vi "Spawn.vi"(7 "ConcreteActor":refnum<class "ConcreteActor.lvclass">) -> (4 "Error":errorcluster, 5 "ConcreteActor":refnum<class "ConcreteActor.lvclass">)   [LabVIEW 2020, in "_Template.lvlib" / "ActorTemplate.lvlib" / "{{Name}}.lvlib" / "ConcreteActor.lvclass"]
uses:
  ConcreteActor.lvclass
  ConcreteActor.lvclass/ConcreteActor.ctl
  jettl/jettl/Actor/Actor.lvclass
panel:
  # "This front panel should not be manipulated."
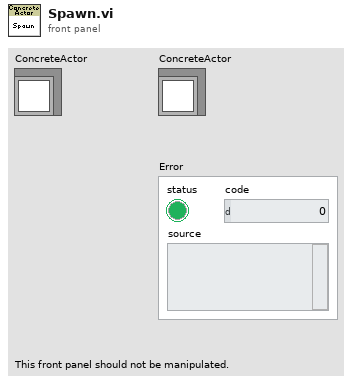
[diagram p1: front panel]
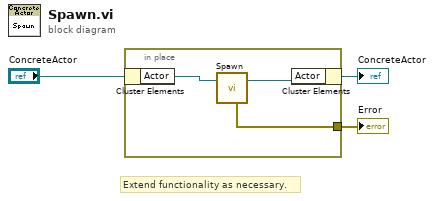
[diagram p0: block diagram]
diagram:
  # "Extend functionality as necessary."
  n1 = in-place {
    in-place-border: [w4] -> w1
    n2 = in-place-cluster #1("ConcreteActor") -> ("Actor"=w6:refnum<class "Actor.lvclass">)
    n3 = call-dynamic "Spawn.vi"("Actor"=w6) -> ("Error"=w4:errorcluster, "Actor"=w5:refnum<class "Actor.lvclass">)  [unwired: 9 in]
    n4 = in-place-cluster #1("Actor"=w5) -> (→"ConcreteActor":refnum<class "ConcreteActor.lvclass">)
  }
  "Error" <- w1
